vi "PQconnect.vi"(8 "error in (no error)":errorcluster, 11 "conninfo":T2={"host"="localhost", "port"="5432", "client_encoding"="WIN1251", "dbname"="data", "user"="postgres", "password"=""}) -> (0 "error out":errorcluster, 2 "PQStatus":T1(ring), 3 "conn":u64)   [LabVIEW 2019, in "libpqutility64.lvlib"]
doc: "Establish PostgreSQL database connection. See PostgreSQL c-lib dokumentation for further information."
uses:
  libpqutility64.lvlib
  ctl/Coninfo.ctl
  libpqlv64/libpqlv64.lvlib
  PostgreSQL.lvlib
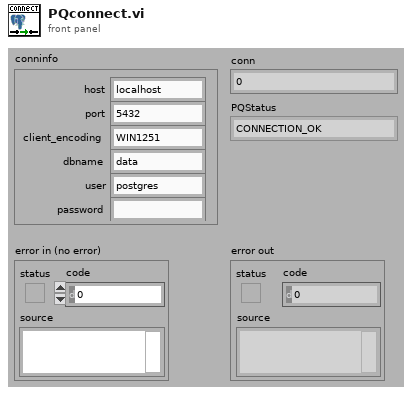
[diagram p1: front panel]
types:
  T1 = enum32{"CONNECTION_OK", "CONNECTION_BAD", "CONNECTION_STARTED", "CONNECTION_MADE", "CONNECTION_AWAITING_RESPONSE", "CONNECTION_AUTH_OK", "CONNECTION_SETENV", "CONNECTION_SSL_STARTUP", "CONNECTION_NEEDED"}
  T2 = typedef "PostgreSQL.lvlib/Coninfo.ctl" = cluster{"host":string, "port":string, "client_encoding":string, "dbname":string, "user":string, "password":string}
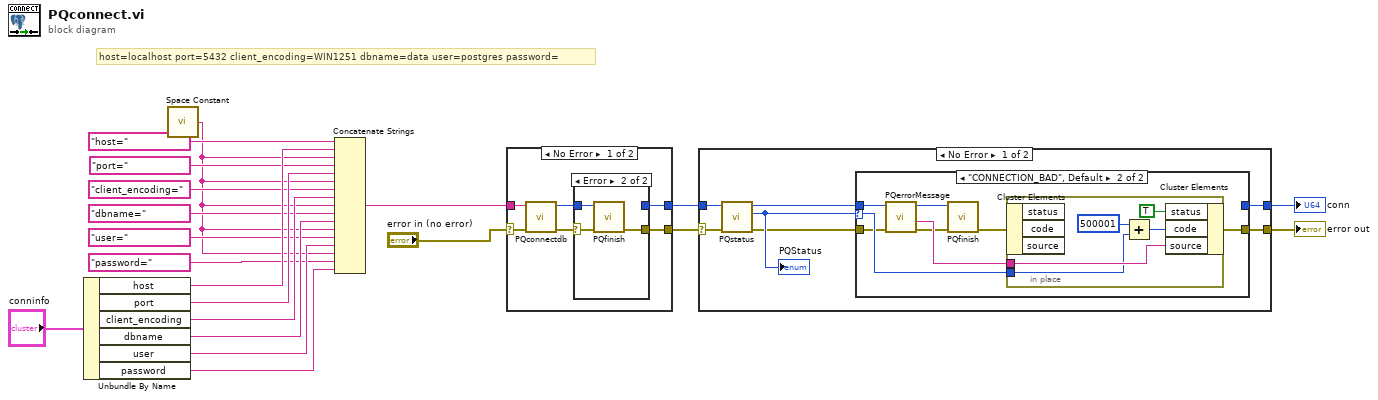
[diagram p0: block diagram]
diagram:
  # "host=localhost port=5432 client_encoding=WIN1251 dbname=data user=postgres password="
  n1 = Unbundle By Name("conninfo") -> ("host"=w13:string, "port"=w11:string, "client_encoding"=w9:string, "dbname"=w7:string, "user"=w5:string, "password"=w2:string)
  n2 = call <vilib>:"Space Constant.vi"() -> ("String"=w4:string)
  n3 = Concatenate Strings("host=" ("string"), w13, w4, "port=" ("string"), w11, w4, "client_encoding=" ("string"), w9, w4, "dbname=" ("string"), w7, w4, "user=" ("string"), w5, w4, "password=" ("string"), w2) -> (w1:string)
  n4 = case shown="No Error" "error in (no error)" {
    selector: "error in (no error)" -> [w25 w32]
    tunnel: w1 -> [w26 _]
    tunnel: [w22 _] -> w18
    tunnel: [w21 w32] -> w19
    frame No Error {
      n5 = call "PQconnectdb.vi"("error in (no error)"=w25, "conninfo"=w26) -> ("error out"=w24:errorcluster, "conn"=w23:u64)  [unwired: 8 in]
      n6 = case shown="Error" w24 {
        selector: w24 -> [w27 w30]
        tunnel: w23 -> [w28 w31]
        tunnel: [w28 _] -> w22
        tunnel: [w27 w29] -> w21
        frame No Error {
        }
        frame Error {
          n7 = call "PQfinish.vi"("error in (no error)"=w30, "conn"=w31) -> ("error out"=w29:errorcluster)  [unwired: 9 in]
        }
      }
    }
    frame Error {
    }
  }
  n8 = case shown="No Error" w19 {
    selector: w19 -> [w34 w56]
    tunnel: w18 -> [w35 w55]
    tunnel: [w38 w55] -> w17
    tunnel: [w39 w56] -> w16
    frame No Error {
      n9 = call "PQstatus.vi"("error in (no error)"=w34, "conn"=w35) -> ("error out"=w33:errorcluster, "PQStatus"=w36:T1, "conn out"=w37:u64)  [unwired: 7 in]
      "PQStatus" <- w36
      n10 = case shown="\"CONNECTION_BAD\", Default" w36 {
        selector: w36 -> [_ w49]
        tunnel: [w40 w48] -> w39
        tunnel: w37 -> [w41 w46]
        tunnel: [w41 _] -> w38
        tunnel: w33 -> [w40 w44]
        frame "CONNECTION_OK" {
        }
        frame "CONNECTION_BAD", Default {
          n11 = call "PQerrorMessage.vi"("error in (no error)"=w44, "conn"=w46) -> ("error out"=w43:errorcluster, "PQerrorMessage"=w47:string, "conn_out"=w45:u64)  [unwired: 7 in]
          n12 = call "PQfinish.vi"("error in (no error)"=w43, "conn"=w45) -> ("error out"=w42:errorcluster)  [unwired: 9 in]
          n13 = in-place {
            in-place-border: w47 -> [w54]
            in-place-border: w49 -> [w51]
            n14 = in-place-cluster #1(w42) -> ()  [unwired: 3 out]
            n15 = Add(x=u32 500001, y=w51) -> (x+y=w50:u32)
            n16 = in-place-cluster #1("status"=TRUE, "code"=w50, "source"=w54) -> (w48:errorcluster)
          }
        }
      }
    }
    frame Error {
    }
  }
  "conn" <- w17
  "error out" <- w16
